vi "NI-Digital History RAM Stream.vi"() -> ()   [LabVIEW 2021]
doc: "Overview\nDemonstrates how to use the History Ram Streaming feature of the NI-Digital Pattern Driver API to capture more samples of history RAM than available memory on the onboard device buffer."
uses:
  <instrlib>/niDigital/niDigital.llb/niDigital Pin State.ctl
  <instrlib>/niDigital/niDigital.llb/niDigital History RAM Cycles to Acquire.ctl
  <instrlib>/niDigital/niDigital.llb/niDigital Load Specifications Levels and Timing (Single).vi
  <instrlib>/niDigital/niDigital.llb/niDigital Burst Pattern (Burst Only).vi
  <instrlib>/niDigital/niDigital.llb/niDigital Get Pattern Pin Names.vi
  <instrlib>/niDigital/niDigital.llb/niDigital Configure Cycle Number History RAM Trigger.vi
  <instrlib>/niDigital/niDigital.llb/niDigital Fetch History RAM Cycle Information (1D Pin States).vi
panel:
  in  "Site":string="site0"
  in  "Pin":string="DUTPin1"
  out "Vector Period (s)":dbl format="%#_6p"
  in  "Simulate?":bool=TRUE
  in  "Resource Name":refnum<k15>="PXI1Slot2,PXI1Slot3" caption="resource name"
  out "Waveform":i16[](graph)
  out "Number of Samples":i64(slide) scale=0.0..100000.0
  in  "Streaming":bool=TRUE
  # "Overview\nDemonstrates how to use the History Ram Streaming feature of the NI-Digital Pattern Driver API to capture more samples of history RAM than available memory on the onboard device buffer.\n\nInstructions\n1. Use the resource name control to select the digital pattern instrument. Ensure that the instrument name in the PinMap.pinmap file matches the resource name of the digital pattern instrument. The default value for the resource name is \"PXI1Slot2,PXI1Slot3\".\n2. Input the Pin and Site of interest into the respective fields. \"DUTPin1\" and \"site0\" are the default values\n3. Uncheck 'Simulate?' and modify the resource name as appropriate. \nImportant: While this example will run in simulation mode without error, no data will be displayed.\n4. Run the VI\n5. Toggle 'Streaming' and re-run the VI. Note that with streaming disabled we fetch all samples available on the onboard buffer at once, while with streaming enabled we can capture all samples in smaller chunks"
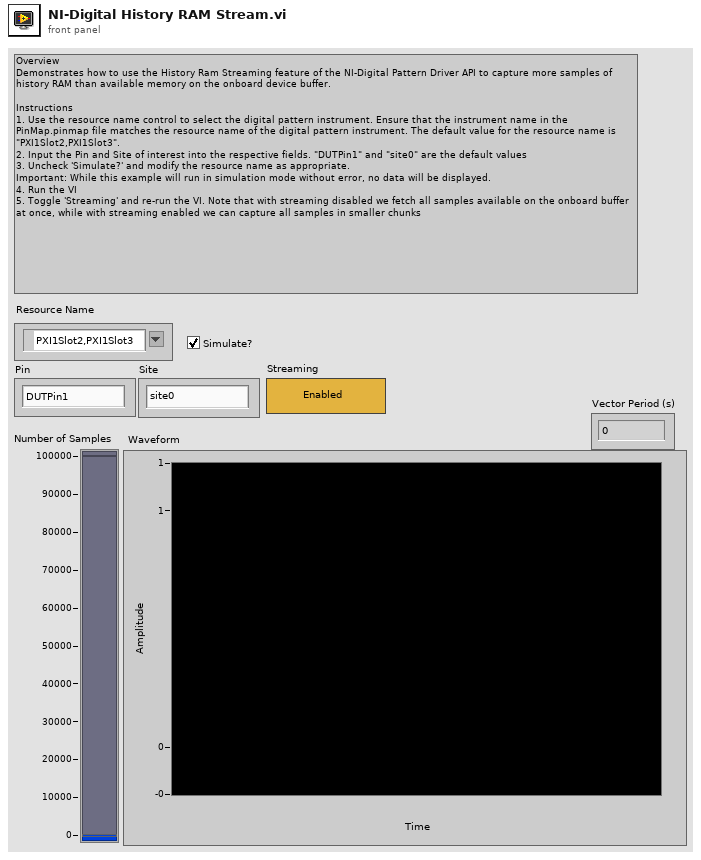
[diagram p1: front panel]
types:
  T1 = typedef "niDigital History RAM Cycles to Acquire.ctl" = i32
  T2 = typedef "niDigital History RAM Cycle Information (1D Pin States).ctl" = cluster{"pattern name":string, "time set name":string, "vector number":i64, "cycle number":i64, "expected pin states":T3[], "actual pin states":T3[], "per pin pass fail":bool[]}
  T3 = typedef "niDigital Pin State.ctl" = u8
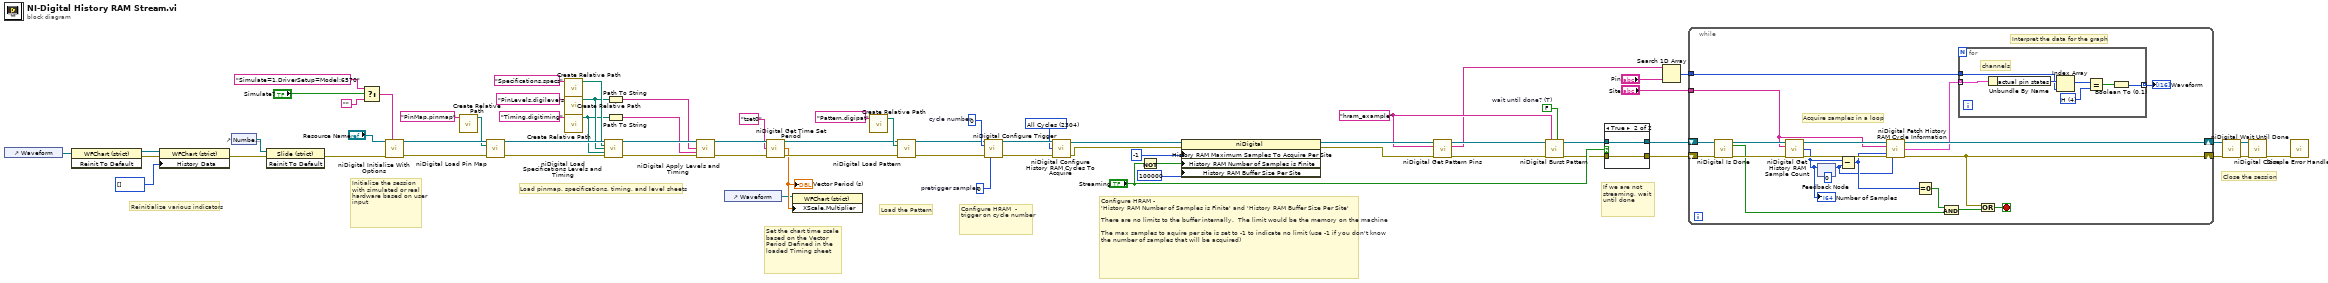
[diagram p0: block diagram]
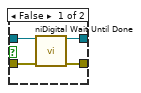
[diagram p2: hidden frame]
diagram:
  w18 = FALSE  # wait until done? (T)
  w2 = "hram_example" ("start label")
  w51 = i64 0  # cycle number
  w52 = T1 2304 items=["Failed Cycles"=2303, "All Cycles"=2304] ("cycles to acquire")
  w53 = 0  # pretrigger samples
  # "Load the Pattern"
  # "Set the chart time scale based on the Vector Period Defined in the loaded Timing sheet"
  # "Load pinmap, specifications, timing, and level sheets"
  # "Reinitialize various indicators"
  # "Close the session"
  # "If we are not streaming, wait until done"
  # "Configure HRAM - \n'History RAM Number of Samples is Finite' and 'History RAM Buffer Size Per Site'\n\nThere are no limits to the buffer internally.  The limit would be the memory on the machine\n\nThe max samples to aquire per site is set to -1 to indicate no limit (use -1 if you don't know the number of samples that will be acquired)"
  # "Configure HRAM  - trigger on cycle number"
  # "Initialize the session with simulated or real hardware based on user input"
  n1 = control-ref of="Waveform"() -> (w17:refnum<vi>)
  n2 = invoke class="WFChart (strict)" method="Reinit To Default"(reference=w17) -> (reference out=w14:refnum<vi>, error out=w16:errorcluster)  [unwired: 2 in, 1 out]
  n3 = property class="WFChart (strict)"(reference=w14, error in=w16, "History Data"=i16[] []) -> (error out=w15:errorcluster)  [unwired: 1 out]
  n4 = control-ref of="Number of Samples"() -> (w55:refnum<vi>)
  n5 = invoke class="Slide (strict)" method="Reinit To Default"(reference=w55, error in=w15) -> (error out=w24:errorcluster)  [unwired: 1 in, 2 out]
  n6 = Select(t="Simulate=1,DriverSetup=Model:6570", s="Simulate?", f="") -> (s? t:f=w29:string)
  n7 = call <instrlib>:"niDigital Initialize With Options.vi"("resource name"="Resource Name", "option string"=w29, "error in"=w24) -> ("instrument handle"=w45:refnum<k15>, "error out"=w44:errorcluster)  [unwired: 11 in]
  n8 = call "Create Relative Path.vi"("file name"="PinMap.pinmap" ("name or relative path")) -> ("appended path"=w39:path)  [unwired: 4 in]
  n9 = call <instrlib>:"niDigital Load Pin Map.vi"("instrument handle"=w45, "pin map file"=w39, "error in"=w44) -> ("instrument handle out"=w42:refnum<k15>, "error out"=w41:errorcluster)  [unwired: 11 in]
  n10 = call "Create Relative Path.vi"("file name"="Specifications.specs" ("name or relative path")) -> ("appended path"=w36:path)  [unwired: 4 in]
  n11 = call "Create Relative Path.vi"("file name"="PinLevels.digilevels" ("name or relative path")) -> ("appended path"=w35:path)  [unwired: 4 in]
  n12 = call "Create Relative Path.vi"("file name"="Timing.digitiming" ("name or relative path")) -> ("appended path"=w34:path)  [unwired: 4 in]
  n13 = call-poly <instrlib>:"niDigital Load Specifications Levels and Timing.vi"("instrument handle"=w42, "specifications file path"=w36, "levels file path"=w35, "timing file path"=w34, "error in"=w41) -> ("instrument handle out"=w50:refnum<k15>, "error out"=w49:errorcluster)  [unwired: 9 in]
  n14 = Path To String(path=w35) -> (string=w43:string)
  n15 = Path To String(path=w34) -> (string=w46:string)
  n16 = call <instrlib>:"niDigital Apply Levels and Timing.vi"("instrument handle"=w50, "levels sheet"=w43, "timing sheet"=w46, "error in"=w49) -> ("instrument handle out"=w21:refnum<k15>, "error out"=w48:errorcluster)  [unwired: 10 in]
  n17 = control-ref of="Waveform"() -> (w12:refnum<vi>)
  n18 = call <instrlib>:"niDigital Get Time Set Period.vi"("instrument handle"=w21, "time set"="tset0", "error in"=w48) -> ("instrument handle out"=w20:refnum<k15>, "period (s)"=w13:dbl, "error out"=w22:errorcluster)  [unwired: 10 in]
  "Vector Period (s)" <- w13
  n19 = property class="WFChart (strict)"(reference=w12, "XScale.Multiplier"=w13) -> ()  [unwired: 1 in, 2 out]
  n20 = call "Create Relative Path.vi"("file name"="Pattern.digipat" ("name or relative path")) -> ("appended path"=w32:path)  [unwired: 4 in]
  n21 = call <instrlib>:"niDigital Load Pattern.vi"("instrument handle"=w20, "pattern file"=w32, "error in"=w22) -> ("instrument handle out"=w26:refnum<k15>, "error out"=w25:errorcluster)  [unwired: 11 in]
  n22 = call-poly <instrlib>:"niDigital Configure Trigger.vi"("instrument handle"=w26, "cycle number"=w51, "error in"=w25, "pretrigger samples"=w53) -> ("instrument handle out"=w69:refnum<k15>, "error out"=w68:errorcluster)  [unwired: 10 in]
  n23 = call <instrlib>:"niDigital Configure History RAM Cycles To Acquire.vi"("instrument handle"=w69, "cycles to acquire"=w52, "error in"=w68) -> ("instrument handle out"=w23:refnum<k15>, "error out"=w62:errorcluster)  [unwired: 11 in]
  n24 = Not(x="Streaming") -> (.not. x?=w60:bool)
  n25 = property on="Property Node" class="niDigital"(reference=w23, error in=w62, "History RAM Maximum Samples To Acquire Per Site"=-1 ("History RAM:Max Samples To Acquire Per Site"), "History RAM Number of Samples is Finite"=w60, "History RAM Buffer Size Per Site"=i64 100000 ("History RAM:Buffer Size Per Site")) -> (reference out=w4:refnum<k15>, error out=w11:errorcluster)
  n26 = call-poly <instrlib>:"niDigital Get Pattern Pins.vi"("instrument handle"=w4, "start label"=w2, "error in"=w11) -> ("instrument handle out"=w3:refnum<k15>, "pin names"=w1:string[], "error out"=w5:errorcluster)  [unwired: 10 in]
  n27 = call-poly <instrlib>:"niDigital Burst Pattern.vi"("instrument handle"=w3, "start label"=w2, "wait until done? (T)"=w18, "error in"=w5) -> ("instrument handle out"=w9:refnum<k15>, "error out"=w57:errorcluster)  [unwired: 10 in]
  n28 = case shown="True" "Streaming" {
    tunnel: w9 -> [w73 w75]
    tunnel: [w72 w75] -> w58
    tunnel: w57 -> [w70 w74]
    tunnel: [w71 w74] -> w56
    frame False {
      n29 = call <instrlib>:"niDigital Wait Until Done.vi"("instrument handle"=w73, "error in"=w70) -> ("instrument handle out"=w72:refnum<k15>, "error out"=w71:errorcluster)  [unwired: 12 in]
    }
    frame True {
    }
  }
  n30 = Search 1D Array(1D array=w1, element="Pin") -> (index of element=w7:i32)  [unwired: 1 in]
  n31 = while {
    shift-right: [w91] -> w66
    shift-left: w58 -> [w92]
    shift-right: [w87] -> w67
    shift-left: w56 -> [w93]
    tunnel: w7 -> [w77]
    tunnel: "Site" -> [w76]
    stop <- w88 stop-if-true
    # "Interpret the data for the graph"
    # "Acquire samples in a loop"
    n32 = call <instrlib>:"niDigital Is Done.vi"("instrument handle"=w92, "error in"=w93) -> ("instrument handle out"=w95:refnum<k15>, "done"=w90:bool, "error out"=w94:errorcluster)  [unwired: 11 in]
    n33 = call <instrlib>:"niDigital Get History RAM Sample Count.vi"("instrument handle"=w95, "site"=w76, "error in"=w94) -> ("instrument handle out"=w83:refnum<k15>, "sample count"=w79:i64, "error out"=w84:errorcluster)  [unwired: 10 in]
    "Number of Samples" <- w79
    n34 = feedback #1(i64 0 ("sample count")) -> (w81:i64)
    n35 = feedback-in #1(w79) -> ()
    n36 = Subtract(x=w79, y=w81) -> (x-y=w82:i64)
    n37 = call-poly <instrlib>:"niDigital Fetch History RAM Cycle Information.vi"("instrument handle"=w83, "site"=w76, "samples to read (-1)"=w82, "error in"=w84, "position"=w81) -> ("instrument handle out"=w91:refnum<k15>, "cycle information"=w86:T2[], "error out"=w87:errorcluster)  [unwired: 8 in]
    n38 = Equal To 0?(x=w82) -> (x = 0?=w85:bool)
    n39 = And(x=w85, y=w90) -> (x .and. y?=w89:bool)
    n40 = for {
      tunnel: w86 -> [w102] mode=indexing
      tunnel: [w97] -> w78 mode=indexing
      tunnel: w77 -> [w96]
      w101 = T3 4 items=["0"=0, "1"=1, "L"=3, "H"=4, "X"=5, "M"=6, "V"=7, "D"=8, "E"=9, "Not A Pin State"=254] ("y")
      # "channels"
      n41 = Unbundle By Name(w102) -> ("actual pin states"=w99:T3[])
      n42 = Index Array(array=w99, index=w96) -> (element=w98:T3)
      n43 = Equal?(x=w98, y=w101) -> (x = y?=w100:bool)
      n44 = Boolean To (0,1)(Boolean=w100) -> (0, 1=w97:i16)
    }
    "Waveform" <- w78
    n45 = Or(x=w87, y=w89) -> (x .or. y?=w88:bool)
  }
  n46 = call <instrlib>:"niDigital Wait Until Done.vi"("instrument handle"=w66, "error in"=w67) -> ("instrument handle out"=w65:refnum<k15>, "error out"=w64:errorcluster)  [unwired: 12 in]
  n47 = call <instrlib>:"niDigital Close.vi"("instrument handle"=w65, "error in"=w64) -> ("error out"=w54:errorcluster)  [unwired: 13 in]
  n48 = call <vilib>:"Simple Error Handler.vi"("error in (no error)"=w54) -> ()  [unwired: 4 in, 5 out]
